vi "Write current state.vi"(8 "error in (no error)":errorcluster, 10 "currentState":u32, 11 "StateManager in":refnum<class "StateManager.lvclass">) -> (0 "error out":errorcluster, 3 "StateManager out":refnum<class "StateManager.lvclass">)   [LabVIEW 2018, in "StateManager.lvclass"]
uses:
  StateManager.lvclass
  StateManager.lvclass/StateManager.ctl
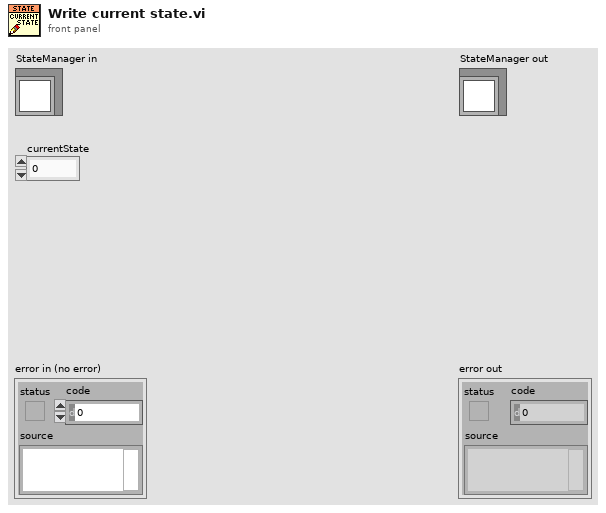
[diagram p1: front panel]
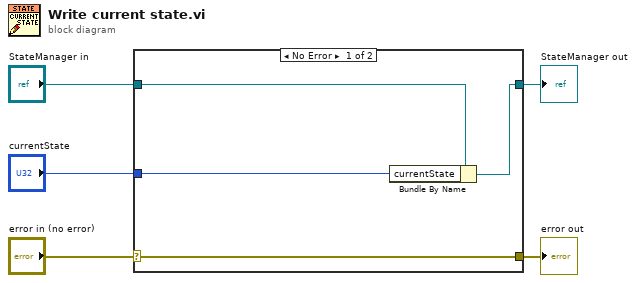
[diagram p0: block diagram]
diagram:
  n1 = case shown="No Error" "error in (no error)" {
    selector: "error in (no error)" -> [w9 w10]
    tunnel: [w9 w10] -> w4
    tunnel: [w7 w11] -> w2
    tunnel: "StateManager in" -> [w8 w11]
    tunnel: "currentState" -> [w6 _]
    frame No Error {
      n2 = Bundle By Name(cluster=w8, "currentState"=w6) -> (w7:refnum<class "StateManager.lvclass">)
    }
    frame Error {
    }
  }
  "error out" <- w4
  "StateManager out" <- w2
